vi "GeneratorTestReport.vi"(8 "error in (no error)":errorcluster caption="错误输入（无错误）", 9 "图表数据in":cluster{i32[], dbl[]}[](array[cluster]), 10 "Record in":string, 11 "路径in":path) -> (0 "error out":errorcluster caption="错误输出")   [LabVIEW 2020]
uses:
  <vilib>/Utility/NIReport.llb/Report Type.ctl
  <vilib>/addons/_office/_exclsub.llb/font.ctl
  <vilib>/Utility/config.llb/Read Key (I32).vi
  <vilib>/Utility/config.llb/Write Key (I32).vi
  <vilib>/Utility/NIReport.llb/NI_report.lvclass
  <vilib>/Utility/NIReport.llb/NI_ReportGenerationCore.lvlib
  <vilib>/addons/_office/NI_ReportGenerationToolkit.lvlib
  <vilib>/Utility/config.llb/NI_LVConfig.lvlib
panel:
  out "工位1_数据图表显示":cluster{i32[], dbl[]}[](graph)
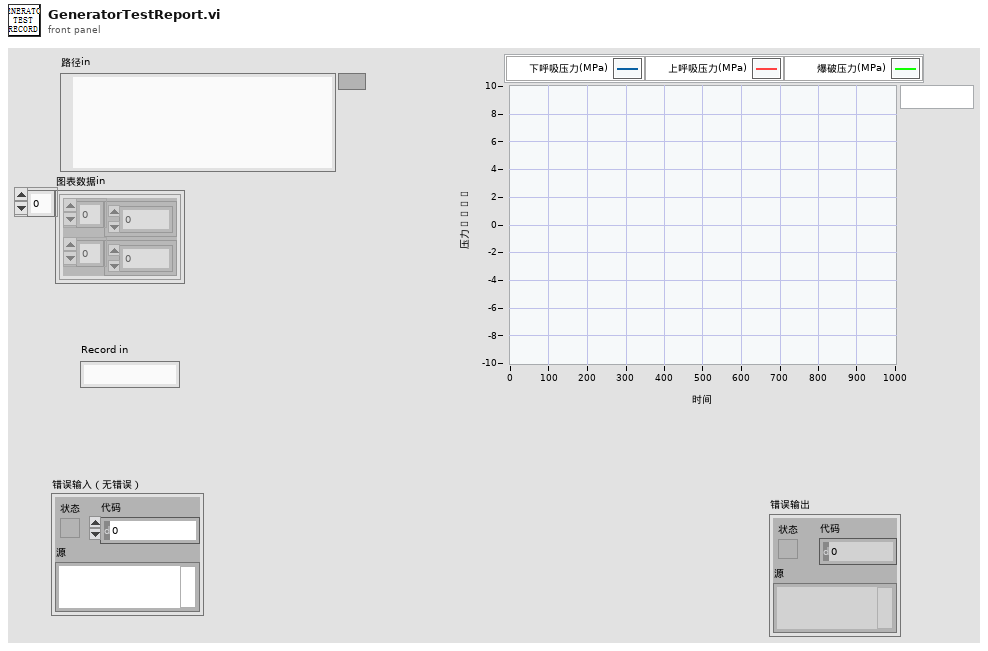
[diagram p1: front panel]
types:
  T1 = typedef "NI_ReportGenerationToolkit.lvlib/font.ctl" = cluster{"font name":string, "font size":dbl, "bold":u16, "italic":u16, "underline":u16, "strike through":u16, "font color":u32}
  T2 = cluster{"position (Excel)":cluster{"row":i32, "column":i32}, "name (Excel)":string, "bookmark (Word)":string}
  T3 = enum16{"maximized", "minimized", "normal", "no change"}
  T4 = typedef "NI_ReportGenerationCore.lvlib/Report Type.ctl" = enum16{"HTML", "Word", "Excel"}
  T5 = typedef "NI_LVConfig.lvlib/Config Data RefNum.ctl" = refnum<k1>
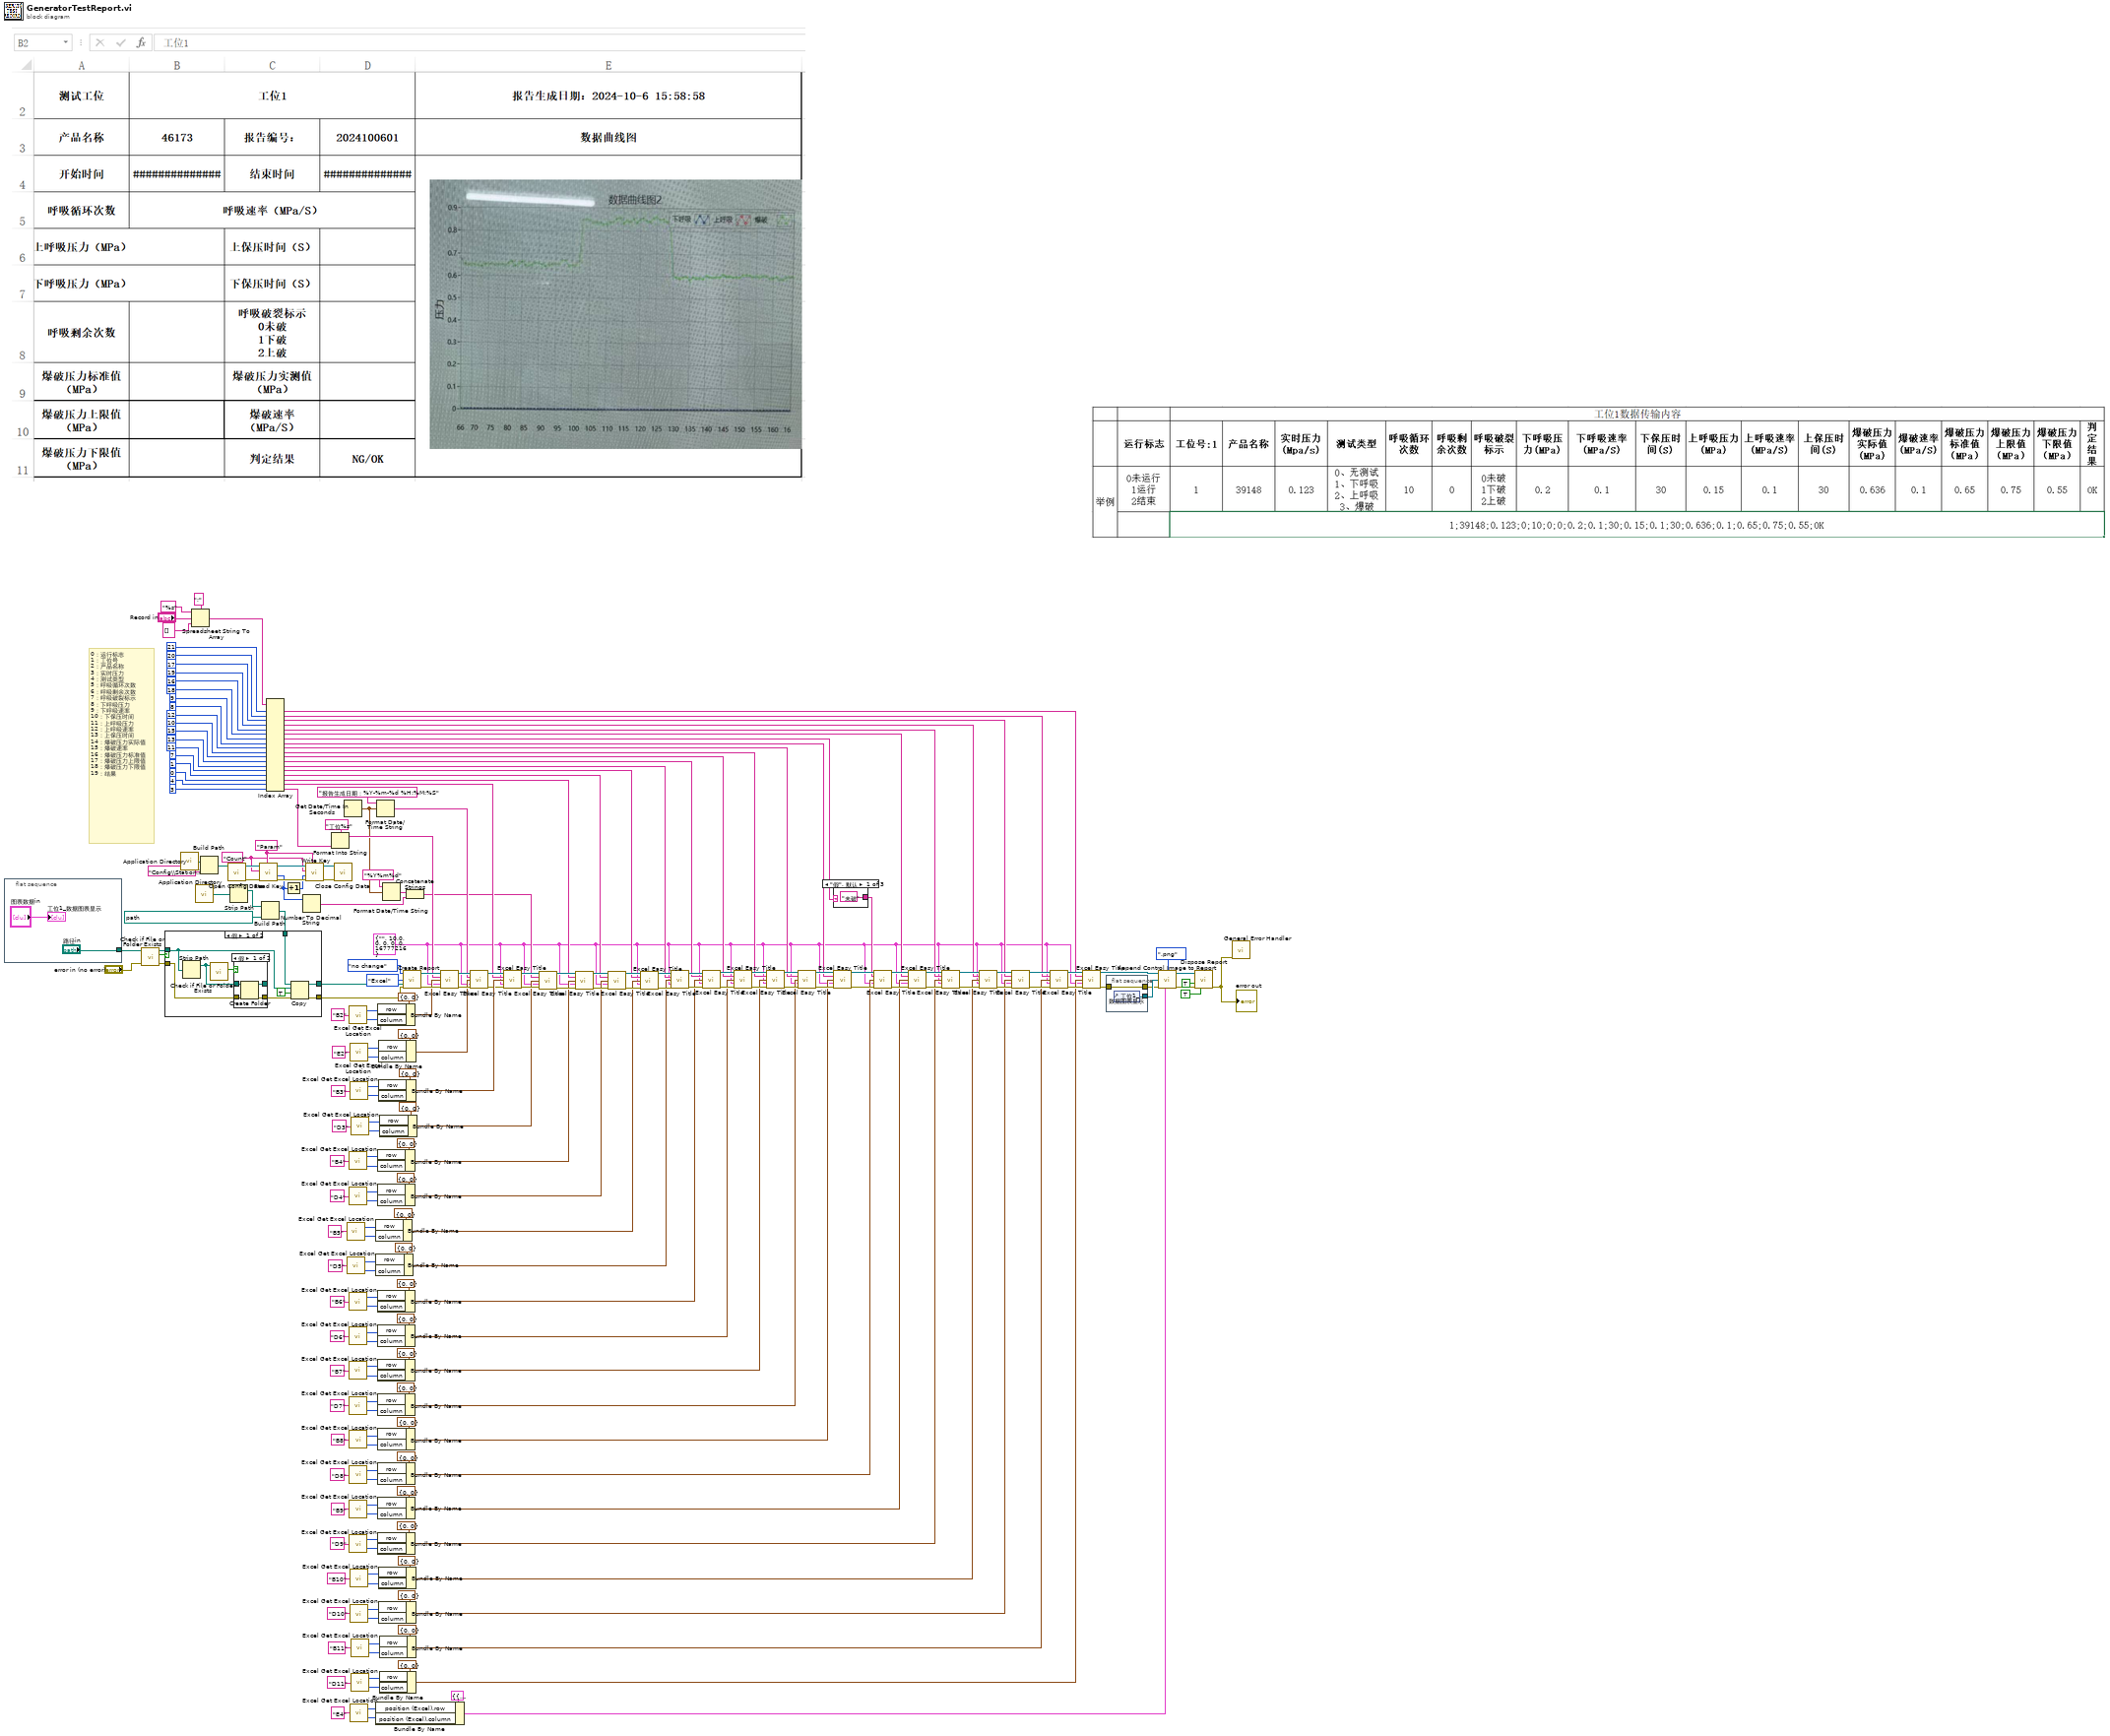
[diagram p0: block diagram]
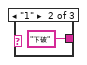
[diagram p2: hidden frame]
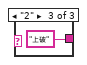
[diagram p3: hidden frame]
diagram:
  w3 = T1 {"font name"="", "font size"=10.0, "bold"=0, "italic"=0, "underline"=0, "strike through"=0, "font color"=16777216} ("font")
  w135 = "Count" ("key")
  w140 = "Param" ("section")
  (unwired) T2 {"position (Excel)"={"row"=0, "column"=0}, "name (Excel)"="", "bookmark (Word)"=""} ("MS Office parameters")
  # "0：运行标志\n1：工位号\n2：产品名称\n3：实时压力\n4：测试类型\n5：呼吸循环次数\n6：呼吸剩余次数\n7：呼吸破裂标示\n8：下呼吸压力\n9：下呼吸速率\n10：下保压时间\n11：上呼吸压力\n12：上呼吸速率\n13：上保压时间\n14：爆破压力实际值\n15：爆破速率\n16：爆破压力标准值\n17：爆破压力上限值\n18：爆破压力下限值\n19：结果"
  n1 = flat-sequence {
    tunnel: ["路径in"] -> w229
    frame #0 {
      "工位1_数据图表显示" <- "图表数据in"
    }
  }
  n2 = call <vilib>:"Check if File or Folder Exists.vi"("error in (no error)"="error in (no error)", "path"=w229) -> ("error out"=w232:errorcluster, "file or folder exists?"=w233:bool, "dup path"=w231:path)  [unwired: 7 in]
  n3 = call <vilib>:"Application Directory.vi"() -> ("Application Directory"=w148:path)
  n4 = Spreadsheet String To Array(delimiter (Tab)=";" ("分隔符(Tab)"), format string="%s" ("格式字符串"), spreadsheet string="Record in", array type (2D Dbl)=string[] []) -> (array=w156:string[])
  n5 = call <vilib>:"Application Directory.vi"() -> ("Application Directory"=w2:path)
  n6 = Build Path(base path=w148, name or relative path="Config\\Station.ini") -> (appended path=w146:path)
  n7 = call <vilib>:"Open Config Data.vi"("configuration file path"=w146) -> ("error out"=w145:errorcluster, "refnum"=w144:T5)  [unwired: 8 in, 1 out]
  n8 = Strip Path(path=w2) -> (stripped path=w1:path)  [unwired: 1 out]
  n9 = call-poly <vilib>:"Read Key.vi"("section"=w140, "error in (no error)"=w145, "key"=w135, "refnum"=w144) -> ("error out"=w138:errorcluster, "value"=w136:i32, "refnum out"=w139:T5)  [unwired: 4 in, 1 out]
  n10 = Build Path(base path=w1, name or relative path=path "Config/呼吸爆破测试报告模板最新.xlsx" ("名称或相对路径")) -> (appended path=w230:path)
  n11 = case shown="假" w233 {
    tunnel: w232 -> [w244 w252]
    tunnel: w231 -> [w236 w251]
    tunnel: [w241 w252] -> w176
    tunnel: w230 -> [w238 _]
    tunnel: [w239 w251] -> w175
    frame False {
      n12 = Strip Path(path=w236) -> (stripped path=w243:path)  [unwired: 1 out]
      n13 = call <vilib>:"Check if File or Folder Exists.vi"("path"=w243) -> ("file or folder exists?"=w242:bool)  [unwired: 8 in, 2 out]
      n14 = case shown="假" w242 {
        tunnel: w244 -> [w248 w250]
        tunnel: [w247 w250] -> w237
        tunnel: w243 -> [w246 w249]
        tunnel: [w245 w249] -> _
        frame False {
          n15 = Create Folder(path (use dialog)=w246, error in=w248) -> (created path=w245:path, error out=w247:errorcluster)  [unwired: 1 in, 1 out]
        }
        frame True {
        }
      }
      n16 = Copy(8:w237, 9:TRUE ("覆盖(F)"), 10:w236, 11:w238) -> (0:w241:errorcluster, 3:w239:path)  [unwired: 1 in, 1 out]
    }
    frame True {
    }
  }
  n17 = Index Array(array=w156, index #1=21 ("索引"), index #2=20 ("索引"), index #3=17 ("索引"), index #4=19 ("索引"), index #5=16 ("索引"), index #6=18 ("索引"), index #7=9 ("索引"), index #8=8 ("索引"), index #9=12 ("索引"), index #10=10 ("索引"), index #11=15 ("索引"), index #12=13 ("索引"), index #13=11 ("索引"), index #14=7 ("索引"), index #15=1 ("索引"), index #16=0 ("索引"), index #17=4 ("索引"), index #18=3 ("索引")) -> (element #1=w5:string, element #2=w6:string, element #3=w23:string, element #4=w24:string, element #5=w41:string, element #6=w42:string, element #7=w59:string, element #8=w60:string, element #9=w75:string, element #10=w76:string, element #11=w91:string, element #12=w104:string, element #13=w112:string, element #14=w115:string, element #15=w124:string, element #16=w131:string, element #17=w151:string, element #18=w147:string)
  n18 = Increment(x=w136) -> (x+1=w137:i32)
  n19 = Number To Decimal String(number=w136) -> (decimal integer string=w142:string)  [unwired: 1 in]
  n20 = call-poly <vilib>:"Write Key.vi"("section"=w140, "error in (no error)"=w138, "value"=w137, "key"=w135, "refnum"=w139) -> ("error out"=w133:errorcluster, "refnum out"=w134:T5)  [unwired: 4 in, 1 out]
  n21 = Format Into String(format string="工位%s" ("格式字符串"), w147) -> (resulting string=w154:string)  [unwired: 2 in, 1 out]
  n22 = call <vilib>:"Close Config Data.vi"("error in (no error)"=w133, "refnum"=w134) -> ()  [unwired: 8 in, 2 out]
  n23 = Get Date/Time In Seconds() -> (seconds since 1Jan1904=w150:timestamp)
  n24 = call <vilib>:"Excel Get Excel Location.vi"("cell's name"="B5") -> ("row"=w118:i32, "column"=w117:i32)
  n25 = call <vilib>:"Excel Get Excel Location.vi"("cell's name"="D5") -> ("row"=w110:i32, "column"=w111:i32)
  n26 = call <vilib>:"Excel Get Excel Location.vi"("cell's name"="B4") -> ("row"=w196:i32, "column"=w195:i32)
  n27 = call <vilib>:"Excel Get Excel Location.vi"("cell's name"="D4") -> ("row"=w127:i32, "column"=w128:i32)
  n28 = call <vilib>:"Excel Get Excel Location.vi"("cell's name"="B6") -> ("row"=w102:i32, "column"=w103:i32)
  n29 = call <vilib>:"Excel Get Excel Location.vi"("cell's name"="D6") -> ("row"=w94:i32, "column"=w93:i32)
  n30 = call <vilib>:"Excel Get Excel Location.vi"("cell's name"="B7") -> ("row"=w80:i32, "column"=w79:i32)
  n31 = call <vilib>:"Excel Get Excel Location.vi"("cell's name"="D7") -> ("row"=w85:i32, "column"=w86:i32)
  n32 = call <vilib>:"Excel Get Excel Location.vi"("cell's name"="B2") -> ("row"=w214:i32, "column"=w213:i32)
  n33 = call <vilib>:"Excel Get Excel Location.vi"("cell's name"="B8") -> ("row"=w73:i32, "column"=w74:i32)
  n34 = call <vilib>:"Excel Get Excel Location.vi"("cell's name"="D8") -> ("row"=w68:i32, "column"=w67:i32)
  n35 = call <vilib>:"Excel Get Excel Location.vi"("cell's name"="B9") -> ("row"=w51:i32, "column"=w50:i32)
  n36 = call <vilib>:"Excel Get Excel Location.vi"("cell's name"="D9") -> ("row"=w56:i32, "column"=w57:i32)
  n37 = call <vilib>:"Excel Get Excel Location.vi"("cell's name"="E2") -> ("row"=w189:i32, "column"=w190:i32)
  n38 = call <vilib>:"Excel Get Excel Location.vi"("cell's name"="B3") -> ("row"=w210:i32, "column"=w211:i32)
  n39 = call <vilib>:"Excel Get Excel Location.vi"("cell's name"="B10") -> ("row"=w39:i32, "column"=w40:i32)
  n40 = call <vilib>:"Excel Get Excel Location.vi"("cell's name"="D10") -> ("row"=w34:i32, "column"=w33:i32)
  n41 = call <vilib>:"Excel Get Excel Location.vi"("cell's name"="E4") -> ("row"=w223:i32, "column"=w222:i32)
  n42 = call <vilib>:"Excel Get Excel Location.vi"("cell's name"="B11") -> ("row"=w12:i32, "column"=w11:i32)
  n43 = call <vilib>:"Excel Get Excel Location.vi"("cell's name"="D11") -> ("row"=w17:i32, "column"=w18:i32)
  n44 = call <vilib>:"Excel Get Excel Location.vi"("cell's name"="D3") -> ("row"=w204:i32, "column"=w203:i32)
  n45 = Bundle By Name(cluster=cluster{"row":i32, "column":i32} {"row"=0, "column"=0} ("start (0, 0)"), "row"=w118, "column"=w117) -> (w116:cluster{"row":i32, "column":i32})
  n46 = Bundle By Name(cluster=T2 {"position (Excel)"={"row"=0, "column"=0}, "name (Excel)"="", "bookmark (Word)"=""} ("MS Office parameters"), "position (Excel).row"=w223, "position (Excel).column"=w222) -> (w221:T2)
  n47 = Bundle By Name(cluster=cluster{"row":i32, "column":i32} {"row"=0, "column"=0} ("start (0, 0)"), "row"=w110, "column"=w111) -> (w107:cluster{"row":i32, "column":i32})
  n48 = Format Date/Time String(time format string (%c)="报告生成日期：%Y-%m-%d %H:%M:%S" ("时间格式字符串(%c)"), seconds (now)=w150) -> (date/time string=w152:string)  [unwired: 1 in]
  n49 = Bundle By Name(cluster=cluster{"row":i32, "column":i32} {"row"=0, "column"=0} ("start (0, 0)"), "row"=w196, "column"=w195) -> (w194:cluster{"row":i32, "column":i32})
  n50 = Bundle By Name(cluster=cluster{"row":i32, "column":i32} {"row"=0, "column"=0} ("start (0, 0)"), "row"=w127, "column"=w128) -> (w123:cluster{"row":i32, "column":i32})
  n51 = Bundle By Name(cluster=cluster{"row":i32, "column":i32} {"row"=0, "column"=0} ("start (0, 0)"), "row"=w102, "column"=w103) -> (w99:cluster{"row":i32, "column":i32})
  n52 = Bundle By Name(cluster=cluster{"row":i32, "column":i32} {"row"=0, "column"=0} ("start (0, 0)"), "row"=w94, "column"=w93) -> (w92:cluster{"row":i32, "column":i32})
  n53 = Bundle By Name(cluster=cluster{"row":i32, "column":i32} {"row"=0, "column"=0} ("start (0, 0)"), "row"=w80, "column"=w79) -> (w78:cluster{"row":i32, "column":i32})
  n54 = Bundle By Name(cluster=cluster{"row":i32, "column":i32} {"row"=0, "column"=0} ("start (0, 0)"), "row"=w85, "column"=w86) -> (w77:cluster{"row":i32, "column":i32})
  n55 = Bundle By Name(cluster=cluster{"row":i32, "column":i32} {"row"=0, "column"=0} ("start (0, 0)"), "row"=w214, "column"=w213) -> (w212:cluster{"row":i32, "column":i32})
  n56 = Bundle By Name(cluster=cluster{"row":i32, "column":i32} {"row"=0, "column"=0} ("start (0, 0)"), "row"=w73, "column"=w74) -> (w62:cluster{"row":i32, "column":i32})
  n57 = Bundle By Name(cluster=cluster{"row":i32, "column":i32} {"row"=0, "column"=0} ("start (0, 0)"), "row"=w68, "column"=w67) -> (w61:cluster{"row":i32, "column":i32})
  n58 = Bundle By Name(cluster=cluster{"row":i32, "column":i32} {"row"=0, "column"=0} ("start (0, 0)"), "row"=w51, "column"=w50) -> (w45:cluster{"row":i32, "column":i32})
  n59 = Bundle By Name(cluster=cluster{"row":i32, "column":i32} {"row"=0, "column"=0} ("start (0, 0)"), "row"=w56, "column"=w57) -> (w44:cluster{"row":i32, "column":i32})
  n60 = Bundle By Name(cluster=cluster{"row":i32, "column":i32} {"row"=0, "column"=0} ("start (0, 0)"), "row"=w189, "column"=w190) -> (w182:cluster{"row":i32, "column":i32})
  n61 = Bundle By Name(cluster=cluster{"row":i32, "column":i32} {"row"=0, "column"=0} ("start (0, 0)"), "row"=w210, "column"=w211) -> (w207:cluster{"row":i32, "column":i32})
  n62 = Bundle By Name(cluster=cluster{"row":i32, "column":i32} {"row"=0, "column"=0} ("start (0, 0)"), "row"=w39, "column"=w40) -> (w28:cluster{"row":i32, "column":i32})
  n63 = Bundle By Name(cluster=cluster{"row":i32, "column":i32} {"row"=0, "column"=0} ("start (0, 0)"), "row"=w34, "column"=w33) -> (w27:cluster{"row":i32, "column":i32})
  n64 = Bundle By Name(cluster=cluster{"row":i32, "column":i32} {"row"=0, "column"=0} ("start (0, 0)"), "row"=w12, "column"=w11) -> (w10:cluster{"row":i32, "column":i32})
  n65 = Bundle By Name(cluster=cluster{"row":i32, "column":i32} {"row"=0, "column"=0} ("start (0, 0)"), "row"=w17, "column"=w18) -> (w9:cluster{"row":i32, "column":i32})
  n66 = Bundle By Name(cluster=cluster{"row":i32, "column":i32} {"row"=0, "column"=0} ("start (0, 0)"), "row"=w204, "column"=w203) -> (w202:cluster{"row":i32, "column":i32})
  n67 = Format Date/Time String(time format string (%c)="%Y%m%d" ("时间格式字符串(%c)"), seconds (now)=w150) -> (date/time string=w143:string)  [unwired: 1 in]
  n68 = call <vilib>:"Create Report.vi"("window state (normal)"=T3."no change", "report type"=Report_Type."Excel", "template (empty)"=w175, "error in (no error)"=w176) -> ("report out"=w220:refnum<class "NI_report.lvclass">, "error out"=w219:errorcluster)  [unwired: 10 in]
  n69 = Concatenate Strings(w143, w142) -> (w141:string)
  n70 = call <vilib>:"Excel Easy Title.vi"("report in"=w220, "title"=w154, "start (0, 0)"=w212, "font"=w3, "error in (no error)"=w219) -> ("report out"=w184:refnum<class "NI_report.lvclass">, "error out"=w186:errorcluster)  [unwired: 8 in, 1 out]
  n71 = call <vilib>:"Excel Easy Title.vi"("report in"=w184, "title"=w152, "start (0, 0)"=w182, "font"=w3, "error in (no error)"=w186) -> ("report out"=w183:refnum<class "NI_report.lvclass">, "error out"=w185:errorcluster)  [unwired: 8 in, 1 out]
  n72 = call <vilib>:"Excel Easy Title.vi"("report in"=w183, "title"=w151, "start (0, 0)"=w207, "font"=w3, "error in (no error)"=w185) -> ("report out"=w218:refnum<class "NI_report.lvclass">, "error out"=w217:errorcluster)  [unwired: 8 in, 1 out]
  n73 = call <vilib>:"Excel Easy Title.vi"("report in"=w218, "title"=w141, "start (0, 0)"=w202, "font"=w3, "error in (no error)"=w217) -> ("report out"=w199:refnum<class "NI_report.lvclass">, "error out"=w200:errorcluster)  [unwired: 8 in, 1 out]
  n74 = call <vilib>:"Excel Easy Title.vi"("report in"=w199, "title"=w131, "start (0, 0)"=w194, "font"=w3, "error in (no error)"=w200) -> ("report out"=w130:refnum<class "NI_report.lvclass">, "error out"=w129:errorcluster)  [unwired: 8 in, 1 out]
  n75 = call <vilib>:"Excel Easy Title.vi"("report in"=w130, "title"=w124, "start (0, 0)"=w123, "font"=w3, "error in (no error)"=w129) -> ("report out"=w122:refnum<class "NI_report.lvclass">, "error out"=w121:errorcluster)  [unwired: 8 in, 1 out]
  n76 = call <vilib>:"Excel Easy Title.vi"("report in"=w122, "title"=w115, "start (0, 0)"=w116, "font"=w3, "error in (no error)"=w121) -> ("report out"=w114:refnum<class "NI_report.lvclass">, "error out"=w113:errorcluster)  [unwired: 8 in, 1 out]
  n77 = call <vilib>:"Excel Easy Title.vi"("report in"=w114, "title"=w112, "start (0, 0)"=w107, "font"=w3, "error in (no error)"=w113) -> ("report out"=w106:refnum<class "NI_report.lvclass">, "error out"=w105:errorcluster)  [unwired: 8 in, 1 out]
  n78 = call <vilib>:"Excel Easy Title.vi"("report in"=w106, "title"=w104, "start (0, 0)"=w99, "font"=w3, "error in (no error)"=w105) -> ("report out"=w98:refnum<class "NI_report.lvclass">, "error out"=w97:errorcluster)  [unwired: 8 in, 1 out]
  n79 = call <vilib>:"Excel Easy Title.vi"("report in"=w98, "title"=w91, "start (0, 0)"=w92, "font"=w3, "error in (no error)"=w97) -> ("report out"=w88:refnum<class "NI_report.lvclass">, "error out"=w87:errorcluster)  [unwired: 8 in, 1 out]
  n80 = call <vilib>:"Excel Easy Title.vi"("report in"=w88, "title"=w76, "start (0, 0)"=w78, "font"=w3, "error in (no error)"=w87) -> ("report out"=w89:refnum<class "NI_report.lvclass">, "error out"=w90:errorcluster)  [unwired: 8 in, 1 out]
  n81 = call <vilib>:"Excel Easy Title.vi"("report in"=w89, "title"=w75, "start (0, 0)"=w77, "font"=w3, "error in (no error)"=w90) -> ("report out"=w64:refnum<class "NI_report.lvclass">, "error out"=w63:errorcluster)  [unwired: 8 in, 1 out]
  n82 = case shown="\"假\", 默认" w59 {
    tunnel: ["未破" "下破" "上破"] -> w58
    frame "假", Default {
    }
    frame "1" {
    }
    frame "2" {
    }
  }
  n83 = call <vilib>:"Excel Easy Title.vi"("report in"=w64, "title"=w60, "start (0, 0)"=w62, "font"=w3, "error in (no error)"=w63) -> ("report out"=w66:refnum<class "NI_report.lvclass">, "error out"=w65:errorcluster)  [unwired: 8 in, 1 out]
  n84 = call <vilib>:"Excel Easy Title.vi"("report in"=w66, "title"=w58, "start (0, 0)"=w61, "font"=w3, "error in (no error)"=w65) -> ("report out"=w47:refnum<class "NI_report.lvclass">, "error out"=w46:errorcluster)  [unwired: 8 in, 1 out]
  n85 = call <vilib>:"Excel Easy Title.vi"("report in"=w47, "title"=w42, "start (0, 0)"=w45, "font"=w3, "error in (no error)"=w46) -> ("report out"=w48:refnum<class "NI_report.lvclass">, "error out"=w49:errorcluster)  [unwired: 8 in, 1 out]
  n86 = call <vilib>:"Excel Easy Title.vi"("report in"=w48, "title"=w41, "start (0, 0)"=w44, "font"=w3, "error in (no error)"=w49) -> ("report out"=w30:refnum<class "NI_report.lvclass">, "error out"=w29:errorcluster)  [unwired: 8 in, 1 out]
  n87 = call <vilib>:"Excel Easy Title.vi"("report in"=w30, "title"=w24, "start (0, 0)"=w28, "font"=w3, "error in (no error)"=w29) -> ("report out"=w32:refnum<class "NI_report.lvclass">, "error out"=w31:errorcluster)  [unwired: 8 in, 1 out]
  n88 = call <vilib>:"Excel Easy Title.vi"("report in"=w32, "title"=w23, "start (0, 0)"=w27, "font"=w3, "error in (no error)"=w31) -> ("report out"=w20:refnum<class "NI_report.lvclass">, "error out"=w19:errorcluster)  [unwired: 8 in, 1 out]
  n89 = call <vilib>:"Excel Easy Title.vi"("report in"=w20, "title"=w6, "start (0, 0)"=w10, "font"=w3, "error in (no error)"=w19) -> ("report out"=w21:refnum<class "NI_report.lvclass">, "error out"=w22:errorcluster)  [unwired: 8 in, 1 out]
  n90 = call <vilib>:"Excel Easy Title.vi"("report in"=w21, "title"=w5, "start (0, 0)"=w9, "font"=w3, "error in (no error)"=w22) -> ("report out"=w201:refnum<class "NI_report.lvclass">, "error out"=w177:errorcluster)  [unwired: 8 in, 1 out]
  n91 = flat-sequence {
    tunnel: [w256] -> w181
    tunnel: w177 -> [w257]
    tunnel: [w257] -> w180
    frame #0 {
      n92 = control-ref of="工位1_数据图表显示"() -> (w256:refnum<vi>)
    }
  }
  n93 = call-dynamic "Append Control Image to Report.vi"("report in"=w201, "image file type (.jpg)"=enum16{".jpg", ".png"}.".png", "ctrl reference"=w181, "error in (no error)"=w180, "MS Office parameters"=w221) -> ("report out"=w193:refnum<class "NI_report.lvclass">, "error out"=w192:errorcluster)  [unwired: 7 in, 2 out]
  n94 = call-dynamic "Dispose Report.vi"("report in"=w193, "save changes? (F)"=TRUE, "error in (no error)"=w192, "close report? (T)"=TRUE) -> ("error out"=w178:errorcluster)  [unwired: 11 in]
  "error out" <- w178
  n95 = call <vilib>:"General Error Handler.vi"("error in (no error)"=w178) -> ()  [unwired: 10 in, 5 out]
